vi "check how many string_0.vi"() -> ()   [LabVIEW 2015]
panel:
  in  "Tab Control":enum32{"Page 1", "Page 2"}(tab)
  out "Totall String":i16
  in  "string":string
  # "Check how many String"
  # "Pardeep Kumar"
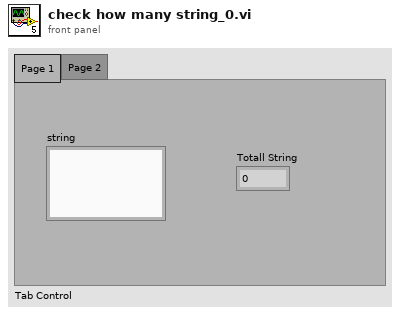
[diagram p1: front panel]
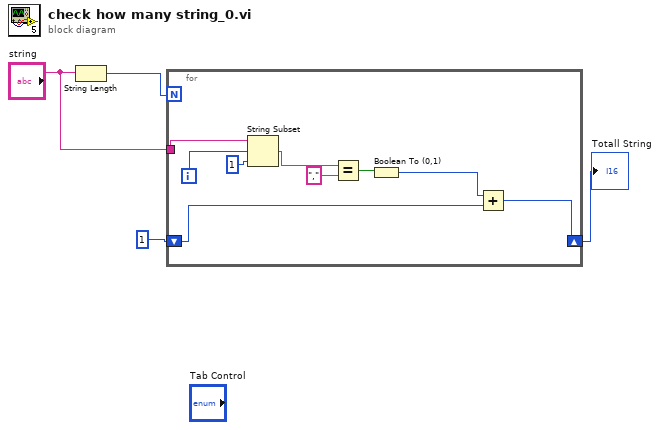
[diagram p0: block diagram]
diagram:
  n1 = String Length(string="string") -> (length=w4:i32)
  n2 = for {
    N: w4 -> [_]
    tunnel: "string" -> [w13]
    shift-right: [w7] -> w2
    shift-left: i16 1 -> [w6]
    i -> [w12]
    n3 = String Subset(string=w13, offset (0)=w12, length (rest)=1 ("length (rest)")) -> (substring=w5:string)
    n4 = Equal?(x=w5, y=",") -> (x = y?=w9:bool)
    n5 = Boolean To (0,1)(Boolean=w9) -> (0, 1=w8:i16)
    n6 = Add(x=w8, y=w6) -> (x+y=w7:i16)
  }
  "Totall String" <- w2
